vi "Auto Current-Amp Based Movement.vi"(8 "Current Based Move Speed":dbl=-0.65, 11 "Movement Angle":dbl=-90.0) -> (0 "Done Moving":bool=TRUE)   [LabVIEW 2017]
panel:
  out "2/13 Pair?":bool
  out "Avg Amp":dbl(graph)=31.1875
  out "PDP 13/14":dbl(graph)=28.625
  out "PDP 1/2":dbl(graph)=33.75
  in  "Amp Threshold":dbl=30.0
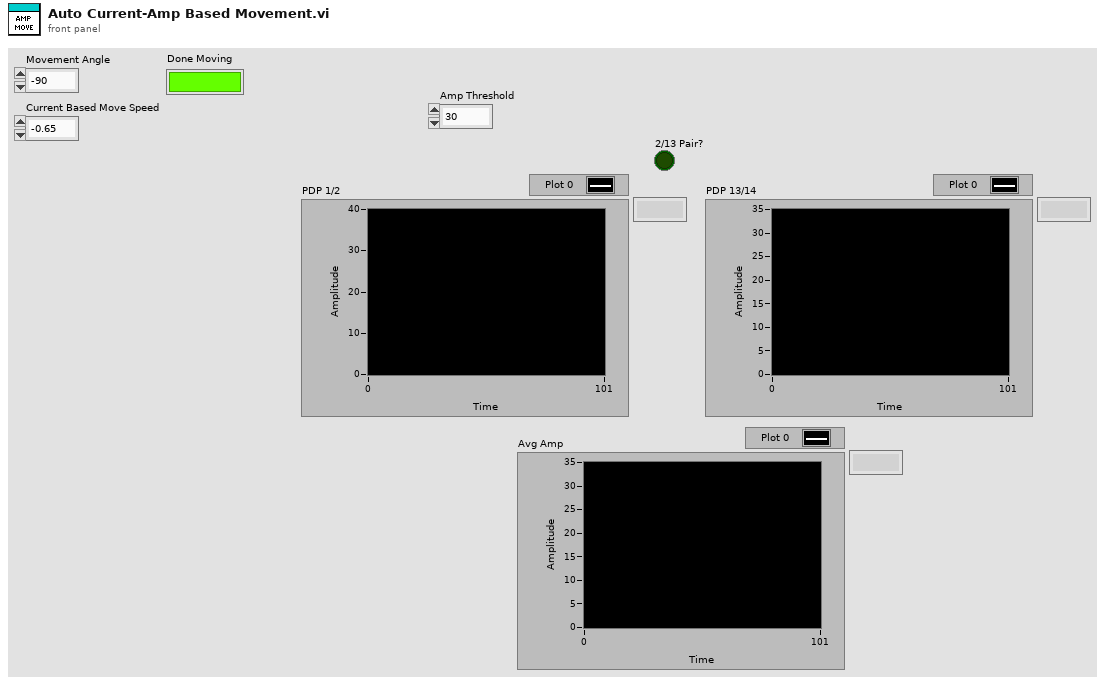
[diagram p1: front panel]
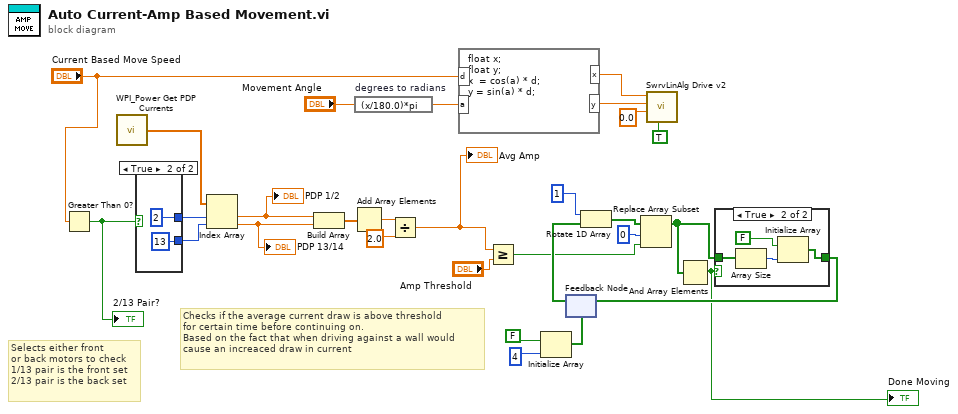
[diagram p0: block diagram]
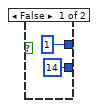
[diagram p2: hidden frame]
diagram:
  # "Selects either front\nor back motors to check\n1/13 pair is the front set\n2/13 pair is the back set"
  # "Checks if the average current draw is above threshold\nfor certain time before continuing on.\nBased on the fact that when driving against a wall would \ncause an increaced draw in current"
  n1 = Greater Than 0?(x="Current Based Move Speed") -> (x > 0?=w1:bool)
  "2/13 Pair?" <- w1
  n2 = call <vilib>:"WPI_Power Get PDP Currents.vi"() -> ("all currents (A)"=w29:dbl[])  [unwired: 13 in, 2 out]
  n3 = case shown="True" w1 {
    tunnel: [1 2] -> w6
    tunnel: [14 13] -> w5
    frame False {
    }
    frame True {
    }
  }
  n4 = Index Array(array=w29, index #1=w6, index #2=w5) -> (element #1=w4:dbl, element #2=w3:dbl)
  "PDP 1/2" <- w4
  "PDP 13/14" <- w3
  n5 = Build Array(w4, w3) -> (w28:dbl[])
  n6 = Add Array Elements(numeric array=w28) -> (sum=w27:dbl)
  n7 = expression code="(x/180.0)*pi" "degrees to radians"("Movement Angle") -> (w25:dbl)
  n8 = Divide(x=w27, y=2.0) -> (x/y=w7:dbl)
  "Avg Amp" <- w7
  n9 = formula code="float x;\nfloat y;\nx  = cos(a) * d;\ny = sin(a) * d;"("d"="Current Based Move Speed", "a"=w25) -> ("x"=w20:dbl, "y"=w21:dbl)
  n10 = Greater Or Equal?(x=w7, y="Amp Threshold") -> (x >= y?=w11:bool)
  n11 = Initialize Array(FALSE, 4 ("dimension size")) -> (w15:bool[])
  n12 = feedback #1(w15) -> (w16:bool[])
  n13 = Rotate 1D Array(1:w16, 2:1 ("n")) -> (0:w18:bool[])
  n14 = Replace Array Subset(array=w18, new element=w11, index=0) -> (w9:bool[])
  n15 = call "SwrvLinAlg Drive v2.vi"("Auto Controls"=TRUE, "Z"=0.0, "Y"=w21, "X"=w20) -> ()  [unwired: 8 in]
  n16 = And Array Elements(Boolean array=w9) -> (logical AND=w8:bool)
  "Done Moving" <- w8
  n17 = case shown="True" w8 {
    tunnel: w9 -> [w34 w36]
    tunnel: [w34 w35] -> w10
    frame False {
    }
    frame True {
      n18 = Array Size(array=w36) -> (size(s)=w37:i32)
      n19 = Initialize Array(FALSE, w37) -> (w35:bool[])
    }
  }
  n20 = feedback-in #1(w10) -> ()
